vi "Test_wait_untill_stopped.vi"() -> ()   [LabVIEW 2019]
panel:
  in  "stop":bool
  out "x .or. y?":bool
  out "Running":bool
  out "Speed 2":i16
  out "Position":i32
  out "Flags 2":T1
  in  "Acceleration":u16
  in  "Speed":i16
  in  "Target":i32
  in  "milliseconds to wait":u32=200
  in  "Address":u8
  out "Flags":T1
  out "Emg stop":bool
  in  "COM Port for serial\nconnection. Check device\nmanager.":string
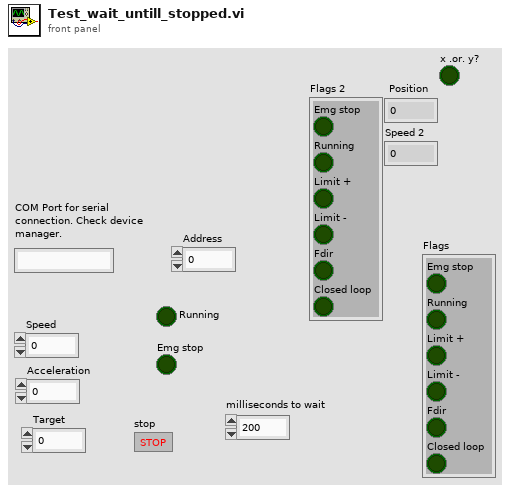
[diagram p1: front panel]
types:
  T1 = cluster{"Emg stop":bool, "Running":bool, "Limit +":bool, "Limit -":bool, "Fdir":bool, "Closed loop":bool}
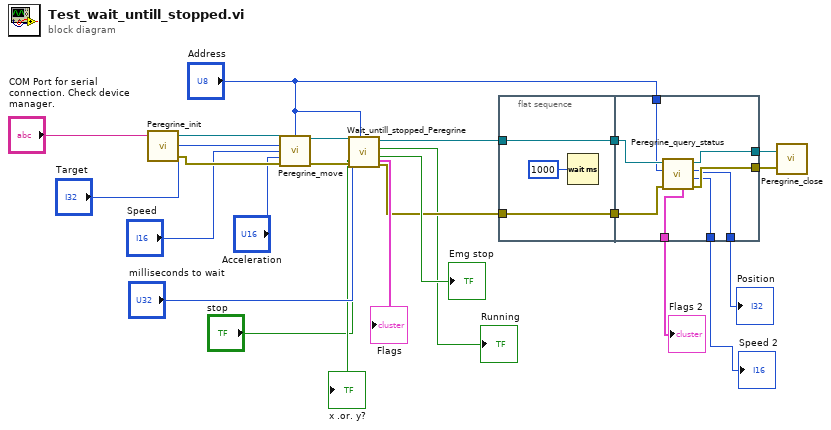
[diagram p0: block diagram]
diagram:
  n1 = call "Peregrine_init.vi"("COM Port for serial\nconnection. Check device\nmanager."="COM Port for serial\nconnection. Check device\nmanager.") -> ("error out"=w22:errorcluster, "Handle out"=w23:refnum<visa-resource-name>)  [unwired: 3 in]
  n2 = call "Peregrine_move.vi"("Handle in"=w23, "Address"="Address", "Target"="Target", "Speed"="Speed", "Acceleration"="Acceleration", "error"=w22) -> ("Handle out"=w21:refnum<visa-resource-name>, "error out"=w20:errorcluster)  [unwired: 8 in]
  n3 = call "Wait_untill_stopped_Peregrine.vi"("Address"="Address", "error"=w20, "stop"="stop", "milliseconds to wait"="milliseconds to wait", "Handle in"=w21) -> ("error out"=w10:errorcluster, "Emg stop"=→"Emg stop":bool, "Running"=→"Running":bool, "Handle out"=w12:refnum<visa-resource-name>, "Flags"=→"Flags":T1, "x .or. y?"=→"x .or. y?":bool)  [unwired: 1 in]
  n4 = flat-sequence {
    tunnel: w12 -> [w26]
    tunnel: [w26] -> w11
    tunnel: w10 -> [w25]
    tunnel: [w25] -> w9
    tunnel: [w35] -> w13
    tunnel: w11 -> [w34]
    tunnel: w9 -> [w33]
    tunnel: [w32] -> w8
    tunnel: [w31] -> w7
    tunnel: "Address" -> [w30]
    tunnel: [w29] -> w5
    tunnel: [w28] -> w4
    frame #0 {
      n5 = Wait (ms)(milliseconds to wait=u32 1000) -> ()  [unwired: 1 out]
    }
    frame #1 {
      n6 = call "Peregrine_query_status.vi"("error"=w33, "Address"=w30, "Handle in"=w34) -> ("error out"=w32:errorcluster, "Speed"=w28:i16, "Position"=w29:i32, "Handle out"=w31:refnum<visa-resource-name>, "Flags"=w35:T1)  [unwired: 4 in]
    }
  }
  n7 = call "Peregrine_close.vi"("error in (no error)"=w8, "Handle in"=w7) -> ()  [unwired: 1 in, 1 out]
  "Flags 2" <- w13
  "Position" <- w5
  "Speed 2" <- w4
